vi "CAN Example.vi"() -> ()   [LabVIEW 2021]
uses:
  src/Typedef/Link Types.ctl
  src/pcap_Parse_Build_CIF.lvclass
  <vilib>/CIF Foundation/CIF Utilities/Time/Time_CIF_U.lvlib
panel:
  out "LabVIEW Time (s)":timestamp
  out "Extended":bool
  out "Remote":bool
  out "ID":u32 format="%.0x"
  out "FD Flags":u8 format="%.0x"
  out "Payload":u8[](array[numeric]) format="%.0x"
  out "File":string
  in  "file path (use dialog)":path
  out "error out":errorcluster
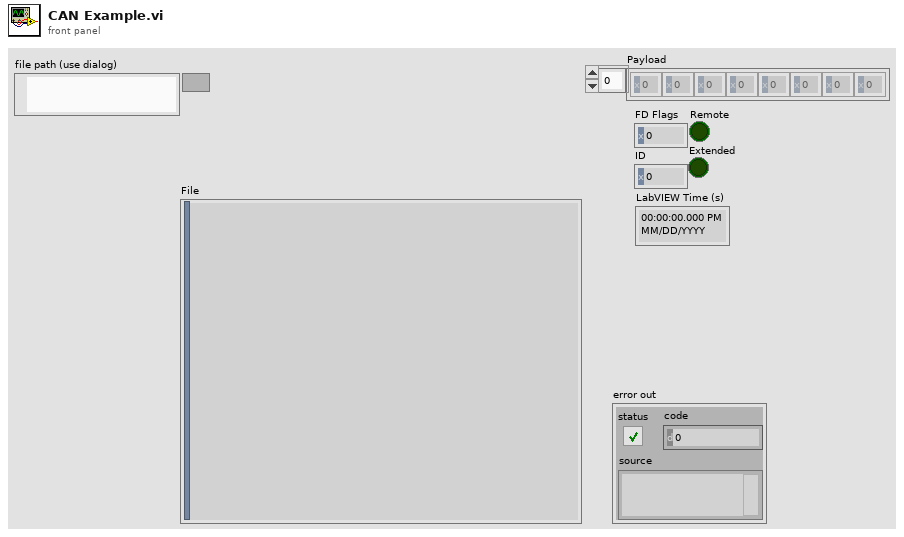
[diagram p1: front panel]
types:
  T1 = typedef "pcap_Parse_Build_CIF.lvclass/Link Types.ctl" = enum16{"Override", "Ethernet", "Socket CAN", "I2C Linux"}
  T2 = enum16{"open", "replace", "create", "open or create", "replace or create", "replace or create with confirmation"}
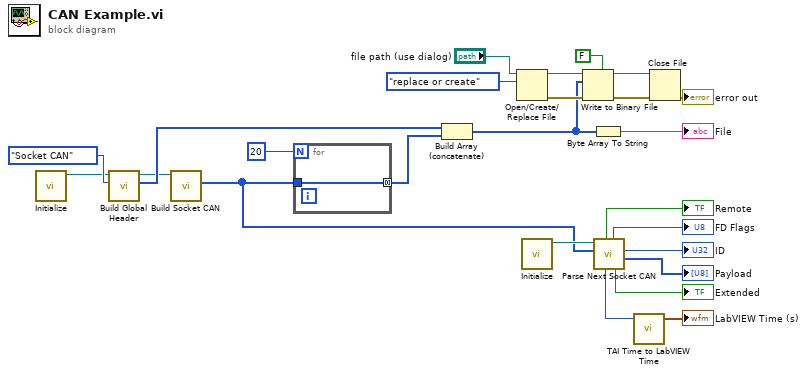
[diagram p0: block diagram]
diagram:
  n1 = call "Initialize.vi"() -> ("pcap Parse and Build out"=w8:refnum<class "pcap_Parse_Build_CIF.lvclass">)  [unwired: 11 in]
  n2 = call "Build Global Header.vi"("Link Types"=Link_Types."Socket CAN", "pcap Parse and Build in"=w8) -> ("Global Header"=w13:u8[], "pcap Parse and Build out"=w11:refnum<class "pcap_Parse_Build_CIF.lvclass">)  [unwired: 7 in, 1 out]
  n3 = call "Build Socket CAN.vi"("pcap Parse and Build in"=w11) -> ("CAN Packet"=w6:u8[])  [unwired: 8 in, 2 out]
  n4 = for {
    N: 20 -> [_]
    tunnel: w6 -> [w26]
    tunnel: [w26] -> w14 mode=concatenating
  }
  n5 = Build Array (concatenate)(w13, w14) -> (w15:u8[])
  n6 = Open/Create/Replace File(file path (use dialog)="file path (use dialog)", operation (0:open)=T2."replace or create") -> (refnum out=w23:refnum<file>, error out=w24:errorcluster)  [unwired: 4 in, 1 out]
  n7 = call "Initialize.vi"() -> ("pcap Parse and Build out"=w7:refnum<class "pcap_Parse_Build_CIF.lvclass">)  [unwired: 11 in]
  n8 = Write to Binary File(file (use dialog)=w23, data=w15, error in=w24, 5:FALSE ("prepend array or string size? (T)")) -> (refnum out=w20:refnum<file>, error out=w19:errorcluster)  [unwired: 2 in, 1 out]
  n9 = Byte Array To String(unsigned byte array=w15) -> (string=→"File":string)
  n10 = call "Parse Next Socket CAN.vi"("CAN pcap in"=w6, "pcap Parse and Build in"=w7) -> ("Payload"=→"Payload":u8[], "ID"=→"ID":u32, "Extended"=→"Extended":bool, "FD Flags"=→"FD Flags":u8, "TAI Time (ns)"=w10:i64, "Remote"=→"Remote":bool)  [unwired: 2 in, 2 out]
  n11 = call <vilib>:"TAI Time to LabVIEW Time.vi"("TAI Time (ns)"=w10) -> ("LabVIEW Time (s)"=→"LabVIEW Time (s)":timestamp)  [unwired: 4 in]
  n12 = Close File(refnum=w20, error in=w19) -> (error out=→"error out":errorcluster)  [unwired: 1 out]
